vi "Init Right Justify.vi"(8 "error in (no error)":errorcluster, 10 "Right Justified Items":refnum<vi>[](array[refnum]), 11 "Splitter Reference":refnum<vi>) -> (0 "error out":errorcluster, 2 "Position Coordinates":cluster{refnum<vi>, i32}[](array[cluster]), 3 "Splitter Reference":refnum<vi>)   [LabVIEW 2013]
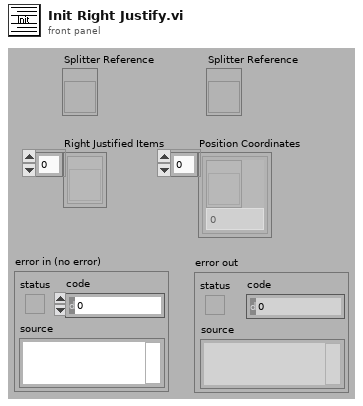
[diagram p1: front panel]
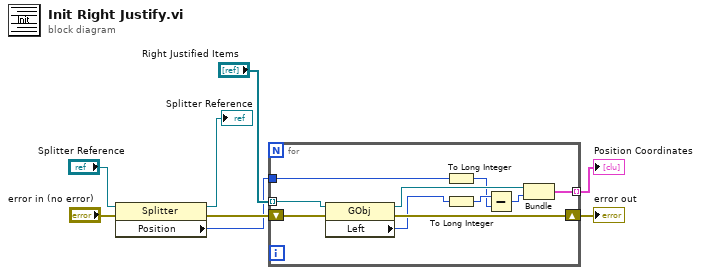
[diagram p0: block diagram]
diagram:
  n1 = property on="Property Node" class="Splitter"(reference="Splitter Reference", error in="error in (no error)") -> (reference out=→"Splitter Reference":refnum<vi>, error out=w3:errorcluster, "Position"=w1:i32)
  n2 = for {
    tunnel: w1 -> [w11]
    tunnel: [w16] -> w8 mode=indexing
    tunnel: "Right Justified Items" -> [w15] mode=indexing
    shift-right: [w13] -> w2
    shift-left: w3 -> [w14]
    n3 = property class="GObj"(reference=w15, error in=w14) -> (reference out=w18:refnum<vi>, error out=w13:errorcluster, "Left"=w9:i32)
    n4 = To Long Integer(number=w11) -> (32bit integer=w10:i32)
    n5 = To Long Integer(number=w9) -> (32bit integer=w12:i32)
    n6 = Subtract(x=w12, y=w10) -> (x-y=w17:i32)
    n7 = Bundle(w18, w17) -> (w16:cluster{refnum<vi>, i32})  [unwired: 1 in]
  }
  "Position Coordinates" <- w8
  "error out" <- w2
